vi "house.vi"() -> ()   [LabVIEW 2014]
panel:
  in  "Thermostat ON/OFF":bool=TRUE
  out "Happiness [%]":dbl(slide) scale=0.0..100.0
  out "Status":string="Water frozen!"
  out "Error":bool
  out "P1":T1
  out "P0":T2
  out "Thermostat [°C]":dbl=20.0
  out "T_out":dbl(slide) scale=-20.0..40.0
  out "Time":timestamp format="%<%H:%M>T"
  in  "VISA resource name":refnum<visa-resource-name>
  out "Device ID":string
  out "Heater temp":dbl(knob) max=60.0 scale=0.0..80.0
  out "Thermometer":dbl(slide) scale=0.0..40.0
  in  "dt":dbl=0.005
  out "Room [°C]":dbl format="%#_3g"
  out "Heater":bool
  in  "Thermostat [°C]":dbl=20.0 min=0.0 max=100.0
  in  "Heater temp [°C]":dbl=50.0 min=0.0 max=80.0 format="%#_2g"
  in  "T_out [°C]":dbl=5.0 min=-200.0 max=100.0
  in  "T_room_0 [°C]":dbl=15.0 min=-40.0 max=100.0
  out "Waveform Chart":cluster{"T_room":dbl, "T_heater":dbl}(graph)
  in  "Stop Button":bool
  # "Thermostat"
  # "Boiler"
  # "System values"
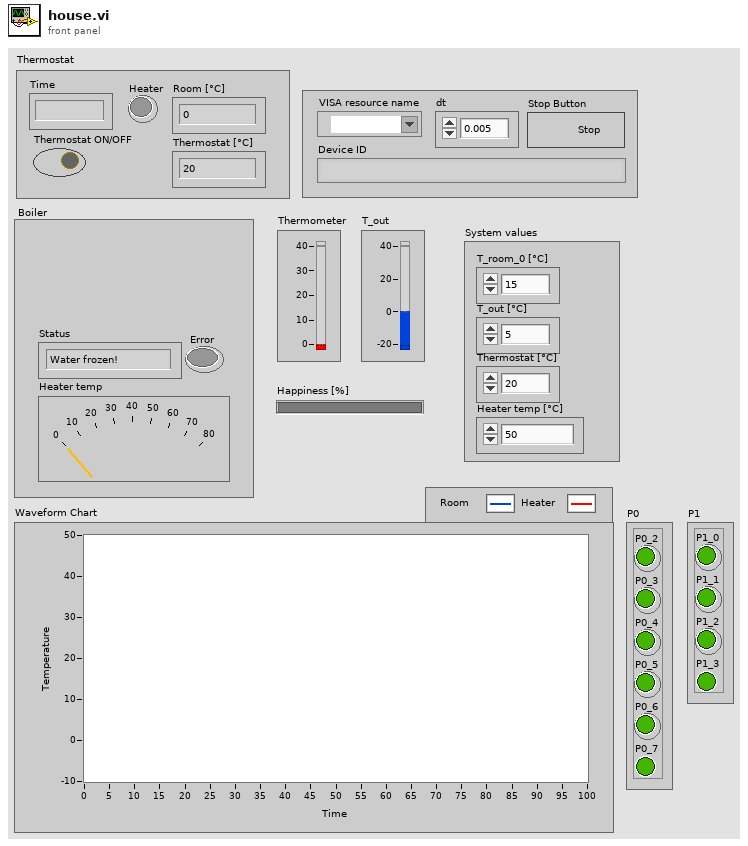
[diagram p1: front panel]
types:
  T1 = cluster{"P1_0":bool, "P1_1":bool, "P1_2":bool, "P1_3":bool, "P1_4":bool, "P1_5":bool, "P1_6":bool, "P1_7":bool, "NC":bool}
  T2 = cluster{"P0_0":bool, "P1_1":bool, "P0_2":bool, "P0_3":bool, "P0_4":bool, "P0_5":bool, "P0_6":bool, "P0_7":bool, "NC":bool}
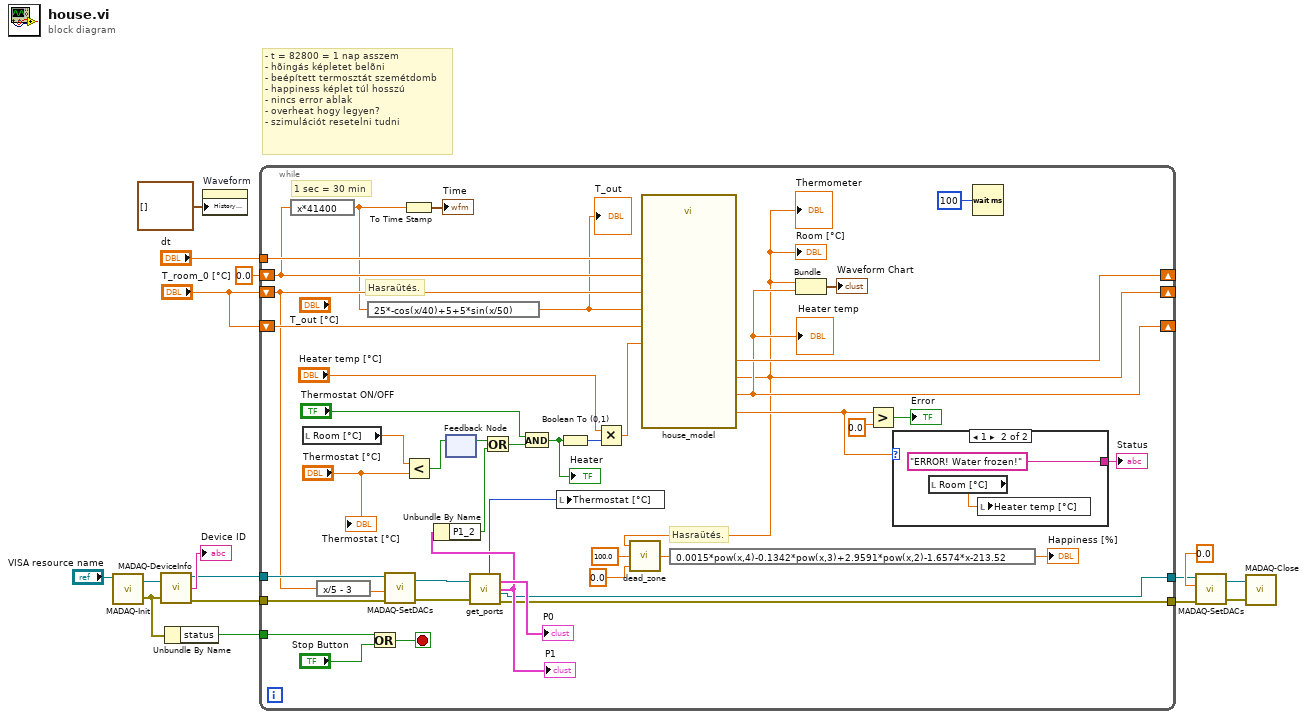
[diagram p0: block diagram]
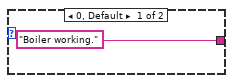
[diagram p2: hidden frame]
diagram:
  # "- t = 82800 = 1 nap asszem\n- hõingás képletet belõni\n- beépített termosztát szemétdomb\n- happiness képlet túl hosszú\n- nincs error ablak\n- overheat hogy legyen?\n- szimulációt resetelni tudni"
  n1 = call "MADAQ-Init.vi"("VISA resource name"="VISA resource name") -> ("error out"=w3:errorcluster, "VISA resource name out"=w11:refnum<visa-resource-name>)  [unwired: 5 in]
  n2 = call "MADAQ-DeviceInfo.vi"("error in (no error)"=w3, "VISA resource name"=w11) -> ("error out"=w10:errorcluster, "Device ID"=→"Device ID":string, "VISA resource name out"=w8:refnum<visa-resource-name>)  [unwired: 3 in]
  n3 = Unbundle By Name(w3) -> ("status"=w2:bool)
  n4 = property on="Waveform" class="WFChart (strict)"("History Data"=cluster{"T_room":dbl, "T_heater":dbl}[] []) -> ()  [unwired: 2 in, 2 out]
  n5 = while {
    shift-right: [w27] -> _
    shift-left: "T_room_0 [°C]" -> [w48]
    shift-right: [w54] -> _
    shift-left: 0.0 ("t") -> [w19]
    shift-right: [w45] -> _
    shift-left: "T_room_0 [°C]" -> [w56]
    tunnel: "dt" -> [w43]
    tunnel: w10 -> [w51]
    tunnel: w8 -> [w50]
    tunnel: [w22] -> w7
    tunnel: w2 -> [w37]
    tunnel: [w23] -> w1
    stop <- w38 stop-if-true
    # "Hasraütés."
    # "Hasraütés."
    # "1 sec = 30 min"
    n6 = expression code="x*41400"(w19) -> (w18:dbl)
    n7 = local read "Room [°C]"() -> (w49:dbl)
    n8 = expression code="x/5 - 3"(w48) -> (w52:dbl)
    n9 = expression code="25*-cos(x/40)+5+5*sin(x/50)"(w18) -> (w17:dbl)
    "T_out" <- w17
    n10 = Or(x=w37, y="Stop Button") -> (x .or. y?=w38:bool)
    n11 = call "MADAQ-SetDACs.vi"("error in (no error)"=w51, "DAC  1 [V]"=w52, "VISA resource name"=w50) -> ("error out"=w46:errorcluster, "VISA resource name out"=w47:refnum<visa-resource-name>)  [unwired: 3 in]
    n12 = To Time Stamp(1:w18) -> (0:→"Time":timestamp)
    n13 = Less?(x=w49, y="Thermostat [°C]") -> (x < y?=w57:bool)
    n14 = feedback #1() -> (w39:bool)  [unwired: 1 in]
    n15 = feedback-in #1(w57) -> ()
    n16 = call "get_ports.vi"("error in (no error)"=w46, "VISA Refnum in"=w47) -> ("error out"=w22:errorcluster, "VISA Refnum out"=w23:refnum<visa-resource-name>, "P1"=w41:T1, "P0"=→"P0":T2, "data"=w21:u8)
    "P1" <- w41
    n17 = Unbundle By Name(w41) -> ("P1_2"=w40:bool)
    n18 = Or(x=w39, y=w40) -> (x .or. y?=w30:bool)
    n19 = And(x="Thermostat ON/OFF", y=w30) -> (x .and. y?=w29:bool)
    "Heater" <- w29
    n20 = local write "Thermostat [°C]"(w21) -> ()
    n21 = Boolean To (0,1)(Boolean=w29) -> (0, 1=w59:i16)
    n22 = Multiply(x="Heater temp [°C]", y=w59) -> (x*y=w55:dbl)
    n23 = call "house_model.vi"("T_out"=w17, "dt"=w43, "t in"=w19, "T_room_0"=w48, "T_heater_0"=w56, "heat_level"=w55) -> ("T_room"=w27:dbl, "error_code"=w33:dbl, "t"=w54:dbl, "T_heater"=w45:dbl)  [unwired: 4 in, 2 out]
    "Room [°C]" <- w27
    "Thermometer" <- w27
    "Heater temp" <- w45
    n24 = call "dead_zone.vi"("min"=0.0, "max"=100.0, "number in"=w27) -> ("number out"=w24:dbl)
    n25 = expression code="0.0015*pow(x,4)-0.1342*pow(x,3)+2.9591*pow(x,2)-1.6574*x-213.52"(w24) -> (→"Happiness [%]":dbl)
    n26 = Bundle("T_room"=w27, "T_heater"=w45) -> (→"Waveform Chart":cluster{"T_room":dbl, "T_heater":dbl})  [unwired: 1 in]
    n27 = Greater?(x=w33, y=0.0) -> (0:→"Error":bool)
    n28 = case shown="1" w33 {
      tunnel: ["Boiler working." "ERROR! Water frozen!"] -> w32
      frame 0, Default {
      }
      frame 1 {
        n29 = local read "Room [°C]"() -> (w62:dbl)
        n30 = local write "Heater temp [°C]"(w62) -> ()
      }
    }
    "Status" <- w32
    n31 = Wait (ms)(milliseconds to wait=u32 100) -> ()  [unwired: 1 out]
    "Thermostat [°C]" <- "Thermostat [°C]"
  }
  n32 = call "MADAQ-SetDACs.vi"("error in (no error)"=w7, "DAC  1 [V]"=0.0, "VISA resource name"=w1) -> ("error out"=w5:errorcluster, "VISA resource name out"=w6:refnum<visa-resource-name>)  [unwired: 3 in]
  n33 = call "MADAQ-Close.vi"("error in (no error)"=w5, "VISA resource name"=w6) -> ()  [unwired: 4 in, 2 out]
